vi "LibXML_GetAllContent.vi"(8 "error in":errorcluster, 10 "xpathexpr":string="/ScanMaster/Devices/Device/description", 11 "doc in":u32) -> (0 "error out":errorcluster, 1 "content list":string[](array[string]), 2 "content":string="the piezo x axis via adwin analog out", 3 "doc copy out":u32, 4 "#ofNodes":u32)   [LabVIEW 2019, in "Tools.lvlib" / "LibXML.lvlib"]
doc: "Get all resolved content in doc at XPath"
uses:
  LibXML.lvlib
  Error Cluster From Error Code_subroutine.vi
  LibXML_IndexNodeList.vi
  LibXML_GetNodeString.vi
  LibXML_GetNodeStrPtr.vi
  LibXML_GetNodeResolvedContentStrPointer.vi
  LibXML_GetStringLength.vi
  LibXML_CopyString.vi
  <vilib>/Utility/error.llb/Trim Whitespace.vi
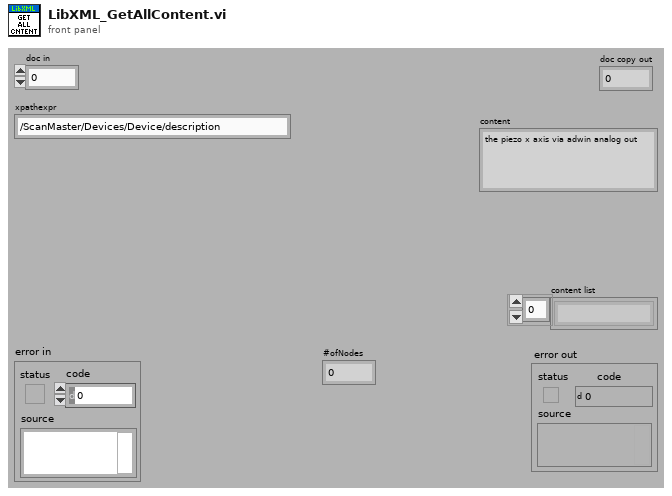
[diagram p1: front panel]
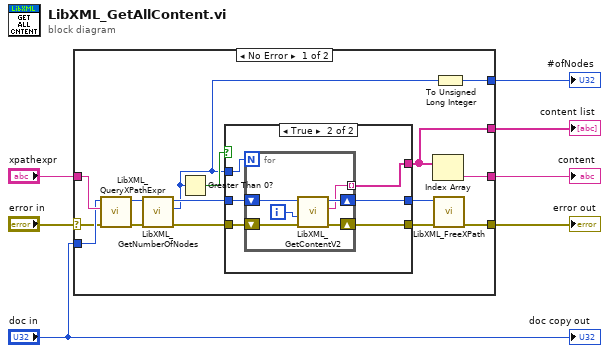
[diagram p0: block diagram]
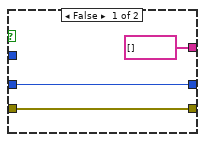
[diagram p2: hidden frame]
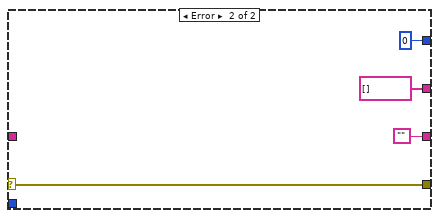
[diagram p3: hidden frame]
diagram:
  n1 = case shown="No Error" "error in" {
    selector: "error in" -> [w9 w41]
    tunnel: "xpathexpr" -> [w20 _]
    tunnel: [w18 ""] -> w6
    tunnel: [w15 string[] []] -> w5
    tunnel: [w8 u32 0 ("#ofNodes")] -> w4
    tunnel: [w12 w41] -> w3
    tunnel: "doc in" -> [w10 _]
    frame No Error {
      n2 = call "LibXML_QueryXPathExpr.vi"("error in"=w9, "XPathExpr"=w20, "doc"=w10) -> ("error out"=w22:errorcluster, "xmlXPathObj"=w19:u32)  [unwired: 7 in]
      n3 = call "LibXML_GetNumberOfNodes.vi"("error in (no error)"=w22, "XPathObj"=w19) -> ("error out"=w21:errorcluster, "#ofNodes"=w14:i32, "XPathObj out"=w17:u32)  [unwired: 7 in]
      n4 = Greater Than 0?(x=w14) -> (x > 0?=w16:bool)
      n5 = case shown="True" w16 {
        tunnel: w21 -> [w25 w31]
        tunnel: w17 -> [w23 w30]
        tunnel: [w25 w29] -> w11
        tunnel: [string[] [] w28] -> w15
        tunnel: w14 -> [_ w27]
        tunnel: [w23 w26] -> w13
        frame False {
        }
        frame True {
          n6 = for {
            N: w27 -> [_]
            shift-right: [w36] -> w29
            shift-left: w31 -> [w35]
            shift-right: [w34] -> w26
            shift-left: w30 -> [w33]
            tunnel: [w32] -> w28 mode=indexing
            i -> [w37]
            n7 = call "LibXML_GetContentV2.vi"("error in"=w35, "index"=w37, "xmlXPathObj"=w33) -> ("error out"=w36:errorcluster, "content"=w32:string, "xmlXPathObj out"=w34:u32)  [unwired: 6 in]
          }
        }
      }
      n8 = Index Array(array=w15) -> (element=w18:string)  [unwired: 1 in]
      n9 = call "LibXML_FreeXPath.vi"("error in"=w11, "XPathObj"=w13) -> ("error out"=w12:errorcluster)  [unwired: 9 in]
      n10 = To Unsigned Long Integer(number=w14) -> (unsigned 32bit integer=w8:u32)
    }
    frame Error {
    }
  }
  "content" <- w6
  "#ofNodes" <- w4
  "error out" <- w3
  "content list" <- w5
  "doc copy out" <- "doc in"
